vi "queue state & data (Array).vi"(6 "Priority State Array? (F)":bool[](array[boolean])=[FALSE], 8 "error in (no error)":errorcluster, 9 "State Data Array":variant[](array[variant]), 10 "State Array":string[](array[string]), 11 "queue in":refnum<queue>) -> (0 "error out":errorcluster, 3 "queue out":refnum<queue>)   [LabVIEW 2024, in "Event-Driven QSM.lvlib"]
doc: "This VI enqueues a list of states into the state machine queue. The states are provided as an array of strings, and each one is enqueued in the order in which it appears in the array. The <b>Priority State Array? (F)</b> input defines whether each individual state should be enqueued at the front (if <b>True</b>) or at the rear (if <b>False</b>) of the queue. This allows combining regular and priority states in a single operation, maintaining full control over the execution order."
uses:
  Event-Driven QSM.lvlib
  state & data--cluster.ctl
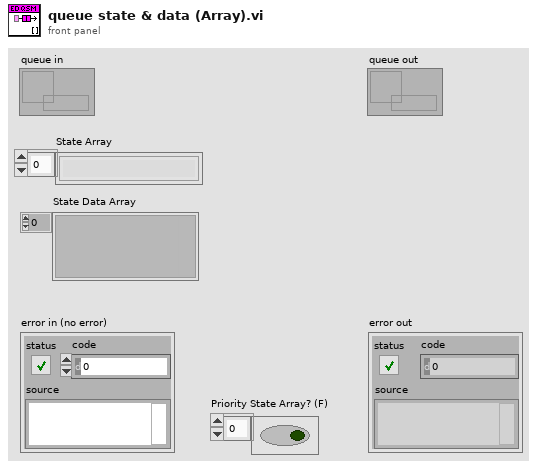
[diagram p1: front panel]
types:
  T1 = typedef "Event-Driven QSM.lvlib/state & data--cluster.ctl" = cluster{"State":string, "Data":variant}
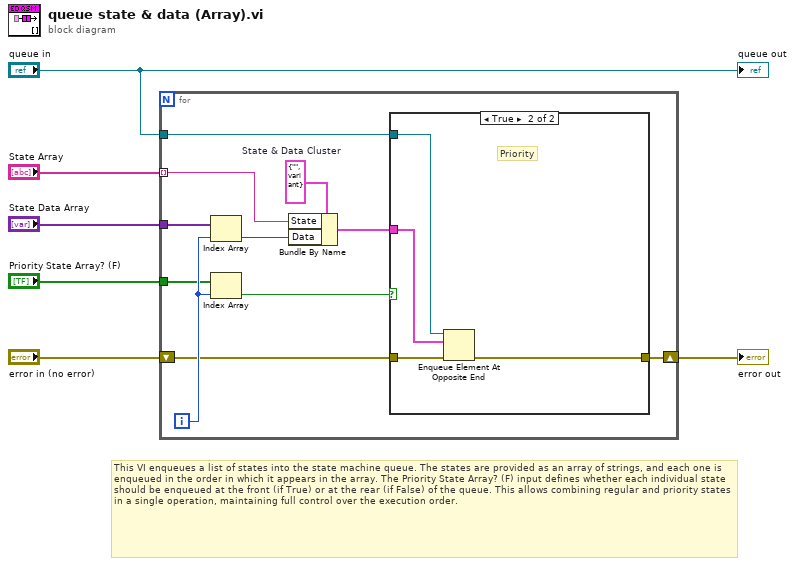
[diagram p0: block diagram]
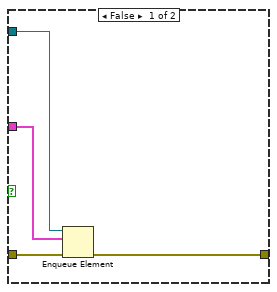
[diagram p2: hidden frame]
diagram:
  # "This VI enqueues a list of states into the state machine queue. The states are provided as an array of strings, and each one is enqueued in the order in which it appears in the array. The Priority State Array? (F) input defines whether each individual state should be enqueued at the front (if True) or at the rear (if False) of the queue. This allows combining regular and priority states in a single operation, maintaining full control over the execution order."
  n1 = for {
    shift-right: [w14] -> w5
    shift-left: "error in (no error)" -> [w16]
    tunnel: "queue in" -> [w15]
    tunnel: "Priority State Array? (F)" -> [w13]
    tunnel: "State Data Array" -> [w11]
    tunnel: "State Array" -> [w10] mode=indexing
    i -> [w17]
    w7 = T1 {"State"="", "Data"=variant}  # State & Data Cluster
    n2 = Index Array(array=w11, index=w17) -> (element=w9:variant)
    n3 = Index Array(array=w13, index=w17) -> (element=w12:bool)
    n4 = Bundle By Name(cluster=w7, "State"=w10, "Data"=w9) -> (w8:T1)
    n5 = case shown="True" w12 {
      tunnel: w16 -> [w21 w25]
      tunnel: w15 -> [w19 w23]
      tunnel: w8 -> [w18 w22]
      tunnel: [w20 w24] -> w14
      frame False {
        n6 = Enqueue Element(queue=w19, element=w18, error in (no error)=w21) -> (error out=w20:errorcluster)  [unwired: 1 in, 2 out]
      }
      frame True {
        # "Priority"
        n7 = Enqueue Element At Opposite End(queue=w23, element=w22, error in (no error)=w25) -> (error out=w24:errorcluster)  [unwired: 1 in, 2 out]
      }
    }
  }
  "error out" <- w5
  "queue out" <- "queue in"
